vi "Get Parameters Test.vi"() -> ()   [LabVIEW 2019]
doc: "This VI allows you to validade that you can get any parameters from the scanner."
uses:
  PF_API.lvclass
panel:
  in  "Parameter Value":string[](array[string])
  in  "Parameter Key":string[](array[string])
  out "body":string
  in  "Scanner IP Address":string
  in  "Host IP Address":string
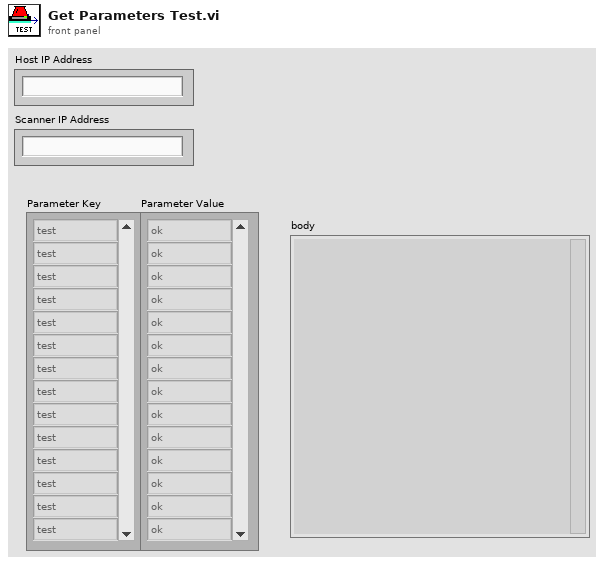
[diagram p1: front panel]
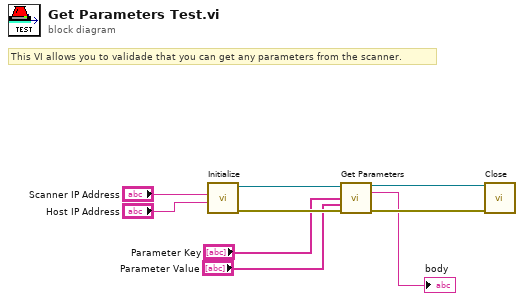
[diagram p0: block diagram]
diagram:
  # "This VI allows you to validade that you can get any parameters from the scanner."
  n1 = call "Initialize.vi"("Host IP Address"="Host IP Address", "Scanner IP Address"="Scanner IP Address") -> ("error out"=w9:errorcluster, "PF_API out"=w5:refnum<class "PF_API.lvclass">)  [unwired: 8 in]
  n2 = call "Get Parameters.vi"("PF_API in"=w5, "Parameter Key"="Parameter Key", "Parameter Value"="Parameter Value", "error in (no error)"=w9) -> ("PF_API out"=w4:refnum<class "PF_API.lvclass">, "body"=→"body":string, "error out"=w6:errorcluster)  [unwired: 9 in]
  n3 = call-dynamic "Close.vi"("error in (no error)"=w6, "PF_API in"=w4) -> ()  [unwired: 8 in, 2 out]
